vi "m1m3_getSample_MirrorForceData.vi"(8 "error in (no error)":errorcluster, 11 "MirrorForceData_Ctl":T1) -> (0 "error out":errorcluster, 2 "function return":i32, 3 "MirrorForceData_Ctl out":T1)   [LabVIEW 2016, in "SALLV_m1m3.lvlib"]
doc: "int m1m3_shm_getSample_MirrorForceDataLV(m1m3_MirrorForceDataLV *MirrorForceData_Ctl );"
uses:
  SALLV_m1m3.lvlib
  DataTypes/MirrorForceData.ctl
  SALLV_m1m3.so
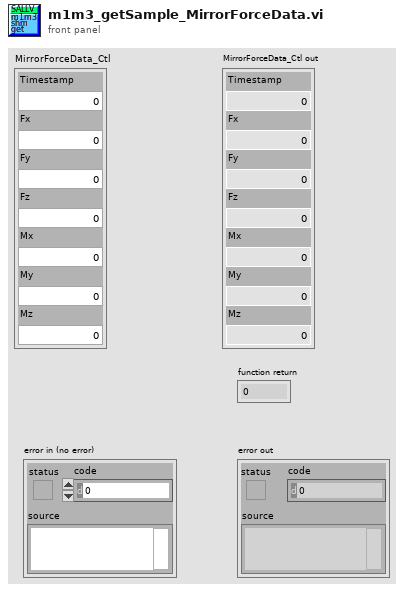
[diagram p1: front panel]
types:
  T1 = typedef "SALLV_m1m3.lvlib/MirrorForceData.ctl" = cluster{"Timestamp":dbl, "Fx":dbl, "Fy":dbl, "Fz":dbl, "Mx":dbl, "My":dbl, "Mz":dbl}
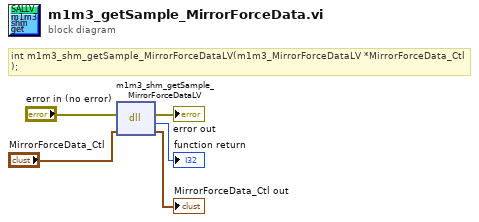
[diagram p0: block diagram]
diagram:
  # "int m1m3_shm_getSample_MirrorForceDataLV(m1m3_MirrorForceDataLV *MirrorForceData_Ctl );"
  n1 = dll-call lib="opt/CODE/SALLV_m1m3/SALLV_m1m3.*" fn="m1m3_shm_getSample_MirrorForceDataLV"(error in="error in (no error)", "MirrorForceData_Ctl"="MirrorForceData_Ctl") -> (error out=→"error out":errorcluster, →"function return":i32, "MirrorForceData_Ctl"=→"MirrorForceData_Ctl out":T1)  [unwired: 2 in, 1 out]
